vi "TestAFM_Driver_Manager.vi"   [LabVIEW 2020, in "AFM_Driver_Manager.lvclass"]
uses:
  AFM_Driver_Manager.lvclass
  <userlib>/LevyLab/Relay Box/Type_defs/Resistor--enum.ctl
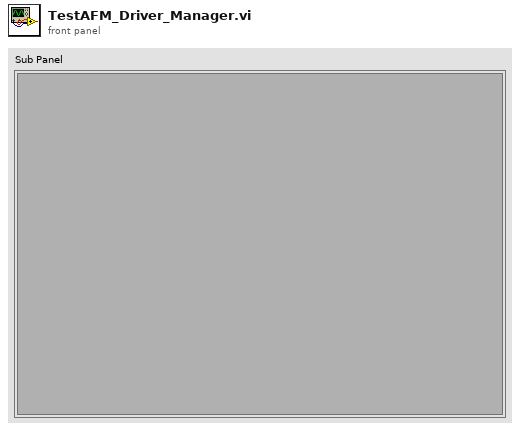
[diagram p1: front panel]
types:
  T1 = typedef "Resistor--enum.ctl" = enum16{"open", "discharge tip", "0 ohms", "100k ohm", "10M ohm", "1G ohm"}
  T2 = cluster{"Name":string, "Litho":cluster{"X":dbl, "Y":dbl, "Speed":dbl, "Voltage":dbl}[], "Set Resistance":T1}[]
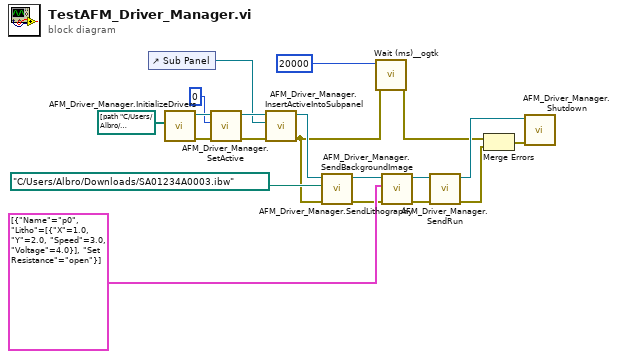
[diagram p0: block diagram]
diagram:
  n1 = control-ref of="Sub Panel"() -> (w15:refnum<vi>)
  n2 = call "AFM_Driver_Manager.InitializeDrivers.vi"("Paths"=path[] [path "C:/Users/Albro/Documents/GitHub/AFM-Lithography/lvsrc/AFMs/Asylum_Driver/Asylum_Driver.vi"]) -> ("error out"=w19:errorcluster, "AFM_Driver_Manager out"=w20:refnum<class "AFM_Driver_Manager.lvclass">)  [unwired: 9 in]
  n3 = call "AFM_Driver_Manager.SetActive.vi"("error in (no error)"=w19, "Active Index"=0, "AFM_Driver_Manager in"=w20) -> ("error out"=w17:errorcluster, "AFM_Driver_Manager out"=w18:refnum<class "AFM_Driver_Manager.lvclass">)  [unwired: 7 in]
  n4 = call "AFM_Driver_Manager.InsertActiveIntoSubpanel.vi"("error in (no error)"=w17, "SubPnl Refnum"=w15, "AFM_Driver_Manager in"=w18) -> ("error out"=w4:errorcluster, "AFM_Driver_Manager out"=w8:refnum<class "AFM_Driver_Manager.lvclass">)  [unwired: 7 in]
  n5 = call "AFM_Driver_Manager.SendBackgroundImage.vi"("error in (no error)"=w4, "Path"=path "C:/Users/Albro/Downloads/SA01234A0003.ibw", "AFM_Driver_Manager in"=w8) -> ("error out"=w5:errorcluster, "AFM_Driver_Manager out"=w7:refnum<class "AFM_Driver_Manager.lvclass">)  [unwired: 7 in]
  n6 = call <userlib>:"Wait (ms)__ogtk.vi"("error in (no error)"=w4, "milliseconds to wait"=u32 20000) -> ("error out"=w2:errorcluster)  [unwired: 8 in, 1 out]
  n7 = call "AFM_Driver_Manager.SendLithography.vi"("error in (no error)"=w5, "Lithography Data"=T2 [{"Name"="p0", "Litho"=[{"X"=1.0, "Y"=2.0, "Speed"=3.0, "Voltage"=4.0}], "Set Resistance"=enum."open"}], "AFM_Driver_Manager in"=w7) -> ("error out"=w11:errorcluster, "AFM_Driver_Manager out"=w12:refnum<class "AFM_Driver_Manager.lvclass">)  [unwired: 7 in]
  n8 = call "AFM_Driver_Manager.SendRun.vi"("error in (no error)"=w11, "AFM_Driver_Manager in"=w12) -> ("error out"=w3:errorcluster, "AFM_Driver_Manager out"=w10:refnum<class "AFM_Driver_Manager.lvclass">)  [unwired: 8 in]
  n9 = Merge Errors(w2, w3) -> (w1:errorcluster)
  n10 = call "AFM_Driver_Manager.Shutdown.vi"("error in (no error)"=w1, "AFM_Driver_Manager in"=w10) -> ()  [unwired: 9 in, 1 out]
